vi "DSF.Engine.Hardware Info.CPU.Set Core Count.vi"(8 "error in (no error)":errorcluster, 10 "Core Count":i32, 11 "CPU Info in":refnum<class "DSF.Engine.Hardware Info.CPU.lvclass">) -> (0 "error out":errorcluster, 3 "CPU Info out":refnum<class "DSF.Engine.Hardware Info.CPU.lvclass">)   [LabVIEW 2017, in "Data Sharing Framework Engine.lvlib" / "DSF.Engine.Hardware Info.CPU.lvclass"]
uses:
  DSF.Engine.Hardware Info.CPU.lvclass
  DSF.Engine.Hardware Info.CPU.lvclass/DSF.Engine.Hardware Info.CPU.ctl
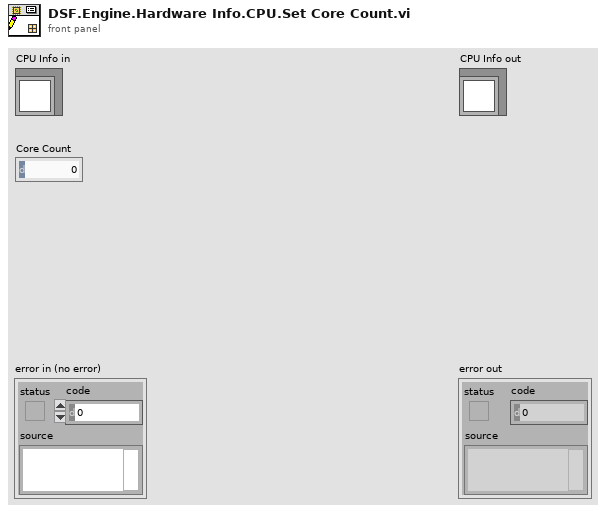
[diagram p1: front panel]
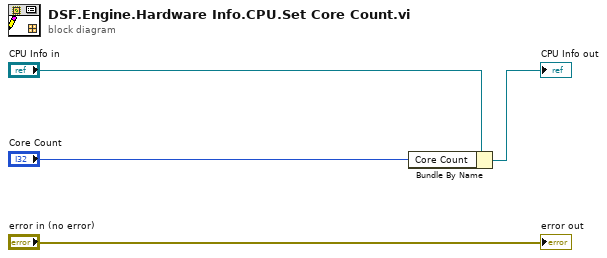
[diagram p0: block diagram]
diagram:
  n1 = Bundle By Name(cluster="CPU Info in", "Core Count"="Core Count") -> (→"CPU Info out":refnum<class "DSF.Engine.Hardware Info.CPU.lvclass">)
  "error out" <- "error in (no error)"
